vi "GetTemp34921T.vi"(3 "error in (no error)":errorcluster) -> (0 "Error out":errorcluster, 1 "String_Temp_34921T":string, 2 "34921A Temp (C)":dbl format="%#.10f")   [LabVIEW 2009]
doc: "Reads the temperature from the probe of the N1911A power meter."
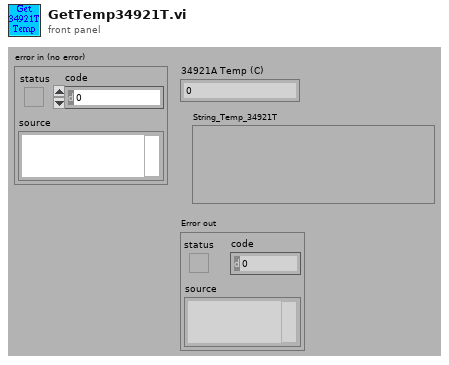
[diagram p1: front panel]
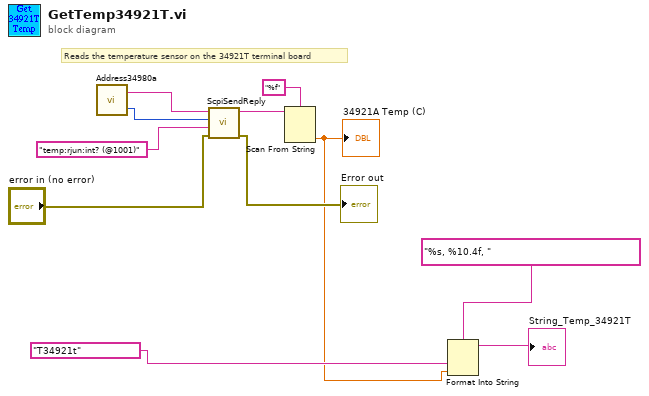
[diagram p0: block diagram]
diagram:
  # "Reads the temperature sensor on the 34921T terminal board"
  n1 = call "Address34980a.vi"() -> ("Port"=w6:i32, "IP address"=w5:string)  [unwired: 2 in]
  n2 = call "ScpiSendReply.vi"("error in (no error)"="error in (no error)", "Command"="temp:rjun:int? (@1001)" ("format string"), "TCP port"=w6, "IP Address"=w5) -> ("Error out"=→"Error out":errorcluster, "Reply"=w9:string)  [unwired: 5 in]
  n3 = Scan From String(format string="%f", input string=w9) -> (output 1=w1:dbl)  [unwired: 3 in, 3 out]
  "34921A Temp (C)" <- w1
  n4 = Format Into String(format string="%s, %10.4f, ", "T34921t", w1) -> (resulting string=→"String_Temp_34921T":string)  [unwired: 2 in, 1 out]
